vi "from string.vi"(8 "error in":errorcluster, 9 "data":string, 10 "version":string, 11 "io configuration in":refnum<class "io configuration.lvclass">) -> (0 "error out":errorcluster, 3 "io configuration out":refnum<class "io configuration.lvclass">)   [LabVIEW 2014, in "io configuration.lvclass"]
doc: "Provides an interface for loading a module configuration from a file or other serialized data source. It is recommended that all children of this class store data in two sets--data required for its own initialization, and any data required for parent initialization--and that each implementation uses the <b>Call Parent Method</b> primitive to de-serialize parent information. As a result, it is expected that every module configuration class calls <b>component configuration.lvclass:From String.vi</b>."
uses:
  io configuration.lvclass
  source/fifo channel/fifo channel.lvclass
  source/fpga channel/fpga channel.lvclass
  <vilib>/NI/Tag Bus Module Framework/channel/TBM channel.lvclass
  io configuration.lvclass/io configuration.ctl
  <vilib>/NI/Tag Bus Module Framework/module configuration/TBM module configuration.lvclass
  <vilib>/NI/Configuration Framework/serializable configuration/NISE_CEF_serializable configuration.lvclass
panel:
  out "associated data":string[](array[string])
  out "discovered subitems":string[](array[string])
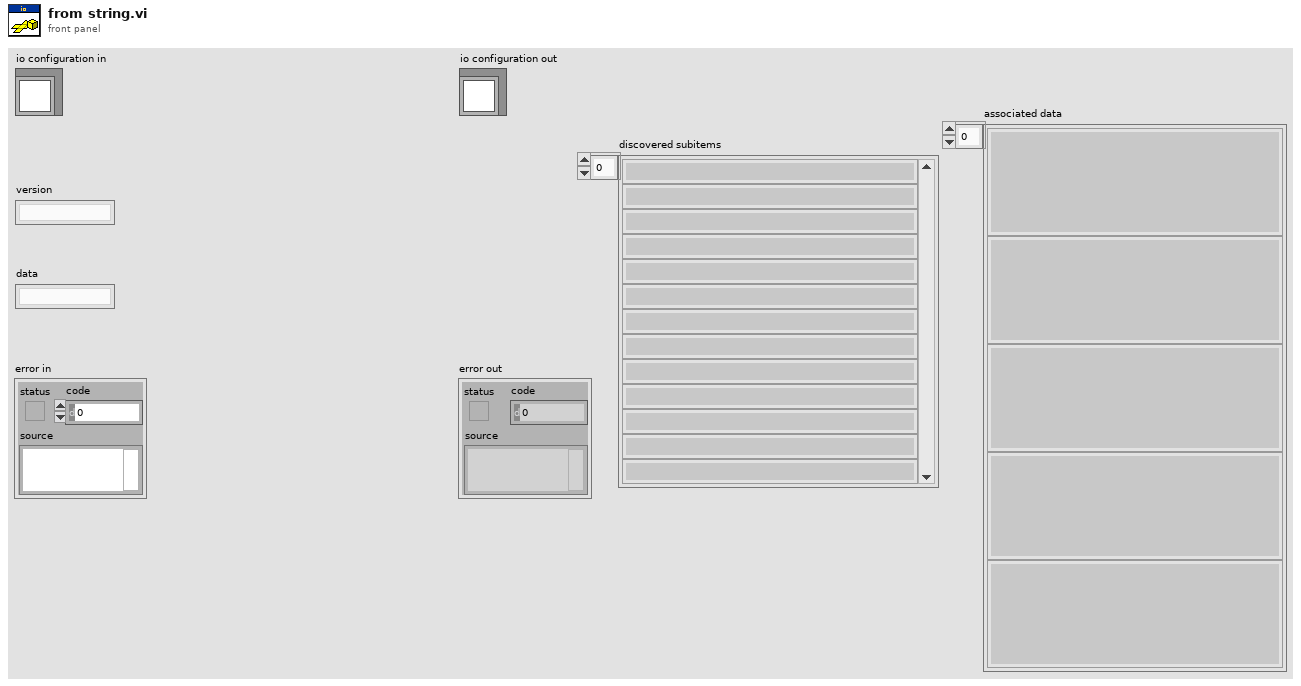
[diagram p1: front panel]
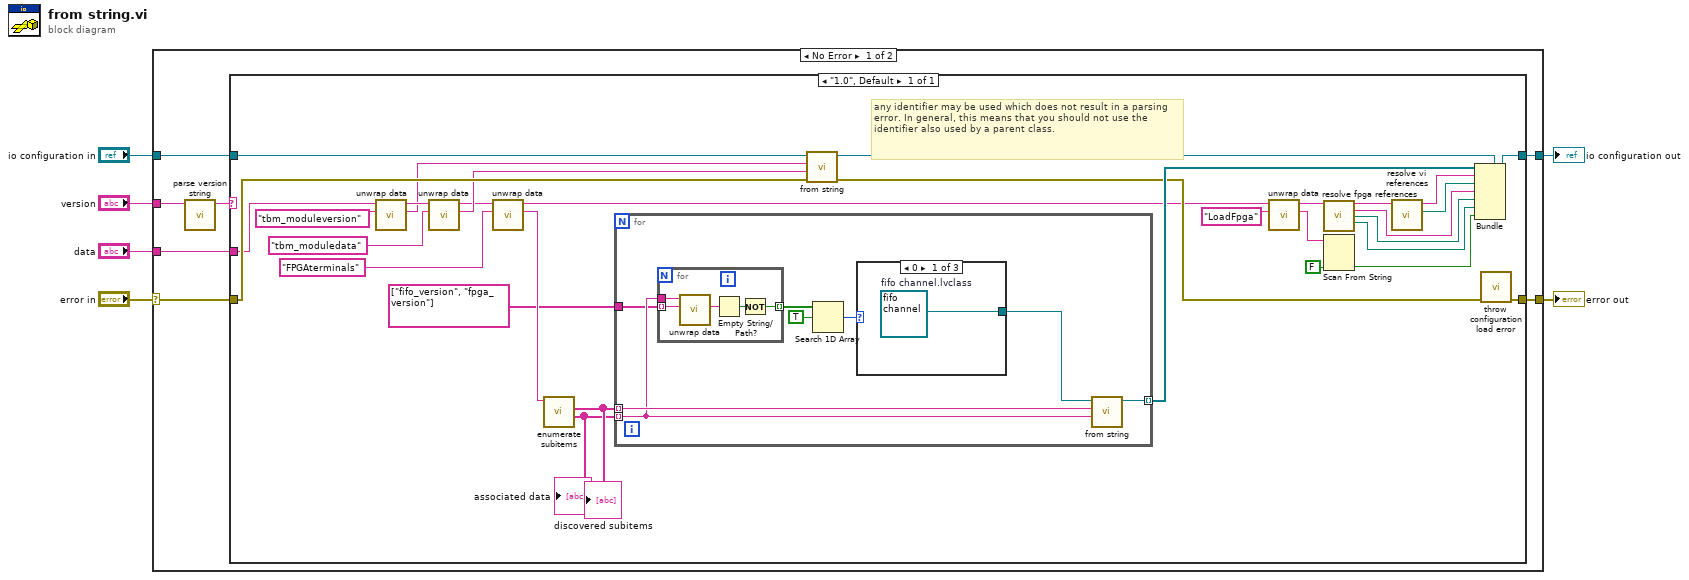
[diagram p0: block diagram]
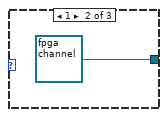
[diagram p2: hidden frame]
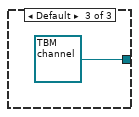
[diagram p3: hidden frame]
diagram:
  n1 = case shown="No Error" "error in" {
    selector: "error in" -> [w7 w62]
    tunnel: "data" -> [w13 _]
    tunnel: "io configuration in" -> [w12 w61]
    tunnel: [w11 w61] -> w5
    tunnel: [w10 w62] -> w4
    tunnel: "version" -> [w9 _]
    frame No Error {
      n2 = call <vilib>:"parse version string.vi"("full version"=w9) -> ("major.minor version"=w8:string)  [unwired: 7 in, 3 out]
      n3 = case shown="\"1.0\", Default" w8 {
        tunnel: w13 -> [w39]
        tunnel: w7 -> [w44]
        tunnel: w12 -> [w43]
        tunnel: [w34] -> w11
        tunnel: [w41] -> w10
        frame "1.0", Default {
          # "any identifier may be used which does not result in a parsing error. In general, this means that you should not use the identifier also used by a parent class."
          n4 = call <vilib>:"unwrap data.vi"("identifier"="tbm_moduleversion" ("additional identifier"), "data to unwrap"=w39) -> ("unwrapped data"=w35:string, "remaining string"=w40:string)  [unwired: 8 in]
          n5 = call <vilib>:"unwrap data.vi"("identifier"="tbm_moduledata" ("additional identifier"), "data to unwrap"=w40) -> ("unwrapped data"=w37:string, "remaining string"=w33:string)  [unwired: 8 in]
          n6 = call <vilib>:"unwrap data.vi"("identifier"="FPGAterminals" ("additional identifier"), "data to unwrap"=w33) -> ("unwrapped data"=w31:string, "remaining string"=w21:string)  [unwired: 8 in]
          n7 = call <vilib>:"enumerate subitems.vi"("data to enumerate"=w31) -> ("associated data"=w29:string[], "discovered subitems"=w30:string[])  [unwired: 8 in, 1 out]
          "discovered subitems" <- w30
          "associated data" <- w29
          n8 = for {
            tunnel: w30 -> [w51] mode=indexing
            tunnel: w29 -> [w49] mode=indexing
            tunnel: [w52] -> w28 mode=indexing
            tunnel: string[] ["fifo_version", "fpga_version"] -> [w48]
            n9 = for {
              tunnel: w49 -> [w57]
              tunnel: [w53] -> w47 mode=indexing
              tunnel: w48 -> [w54] mode=indexing
              n10 = call <vilib>:"unwrap data.vi"("identifier"=w54, "data to unwrap"=w57) -> ("unwrapped data"=w56:string)  [unwired: 8 in, 1 out]
              n11 = Empty String/Path?(string/path=w56) -> (empty?=w55:bool)
              n12 = Not(x=w55) -> (.not. x?=w53:bool)
            }
            n13 = Search 1D Array(1D array=w47, element=TRUE) -> (index of element=w45:i32)  [unwired: 1 in]
            n14 = case shown="0" w45 {
              tunnel: [w58 refnum<class "fpga channel.lvclass"> refnum ("Fxp Channel.lvclass") refnum<class "TBM channel.lvclass"> refnum ("channel")] -> w50
              frame 0 {
                w58 = refnum<class "fifo channel.lvclass"> refnum  # fifo channel.lvclass
              }
              frame 1 {
              }
              frame Default {
              }
            }
            n15 = call-dynamic "from string.vi"("channel data"=w49, "identifier"=w51, "channel in"=w50) -> ("channel out"=w52:refnum<class "TBM channel.lvclass">)  [unwired: 7 in, 1 out]
          }
          n16 = call-parent "from string.vi"("error in"=w44, "data"=w37, "version"=w35, "module configuration in"=w43) -> ("error out"=w27:errorcluster, "module configuration out"=w42:refnum<class "io configuration.lvclass">)  [unwired: 6 in]
          n17 = call <vilib>:"unwrap data.vi"("identifier"="LoadFpga" ("additional identifier"), "data to unwrap"=w21) -> ("unwrapped data"=w17:string, "remaining string"=w19:string)  [unwired: 8 in]
          n18 = call "resolve fpga references.vi"("data to unwrap"=w19) -> ("remaining string"=w24:string, "ResourceName"=w23:string, "Bitfile path"=w22:path, "Bitfile Exe Dir"=w16:path)  [unwired: 11 in]
          n19 = Scan From String(input string=w17, default 1=FALSE ("add enable channel")) -> (output 1=w15:bool)  [unwired: 3 in, 3 out]
          n20 = call "resolve vi references.vi"("remaining string"=w24) -> ("VI path"=w25:path, "VI name"=w26:string)  [unwired: 9 in]
          n21 = Bundle(cluster=w42, w28, w26, w25, w23, w22, w16, w15) -> (w34:refnum<class "io configuration.lvclass">)
          n22 = call <vilib>:"throw configuration load error.vi"("error in"=w27) -> ("error out"=w41:errorcluster)  [unwired: 10 in]
        }
      }
    }
    frame Error {
    }
  }
  "error out" <- w4
  "io configuration out" <- w5
